vi "TestVision_v2.vi"() -> ()   [LabVIEW 2019]
uses:
  <vilib>/vision/Image Controls.llb/IMAQ Image.ctl
  <vilib>/userDefined/High Color/IMAQdx.ctl
  <vilib>/vision/driver/NI_Vision_Acquisition_Software.lvlib
  <vilib>/vision/NI_Vision_Development_Module.lvlib
panel:
  in  "Image Type":T1 items=["Grayscale (U8)", "Grayscale (I16)", "Grayscale (SGL)", "Complex (CSG)", "RGB (U32)", "HSL (U32)", "RGB (U64)", "Grayscale (U16)"]
  out "Circle Found":bool
  out "Fitted Circle":T2 {"Average SNR (dB)" format="%.2f"; "Average Strength" format="%.2f"; "Roundness (Real-World)" format="%.2f"; "Radius (Real-World)" format="%.2f"; "Center (Real-World)"."Y" format="%.2f"; "Center (Real-World)"."X" format="%.2f"; "Radius (Pixels)" format="%.2f"; "Center (Pixels)"."Y" format="%.2f"; "Center (Pixels)"."X" format="%.2f"}
  out "Image Out":T3
  out "Image 2":T3(plugin-control)
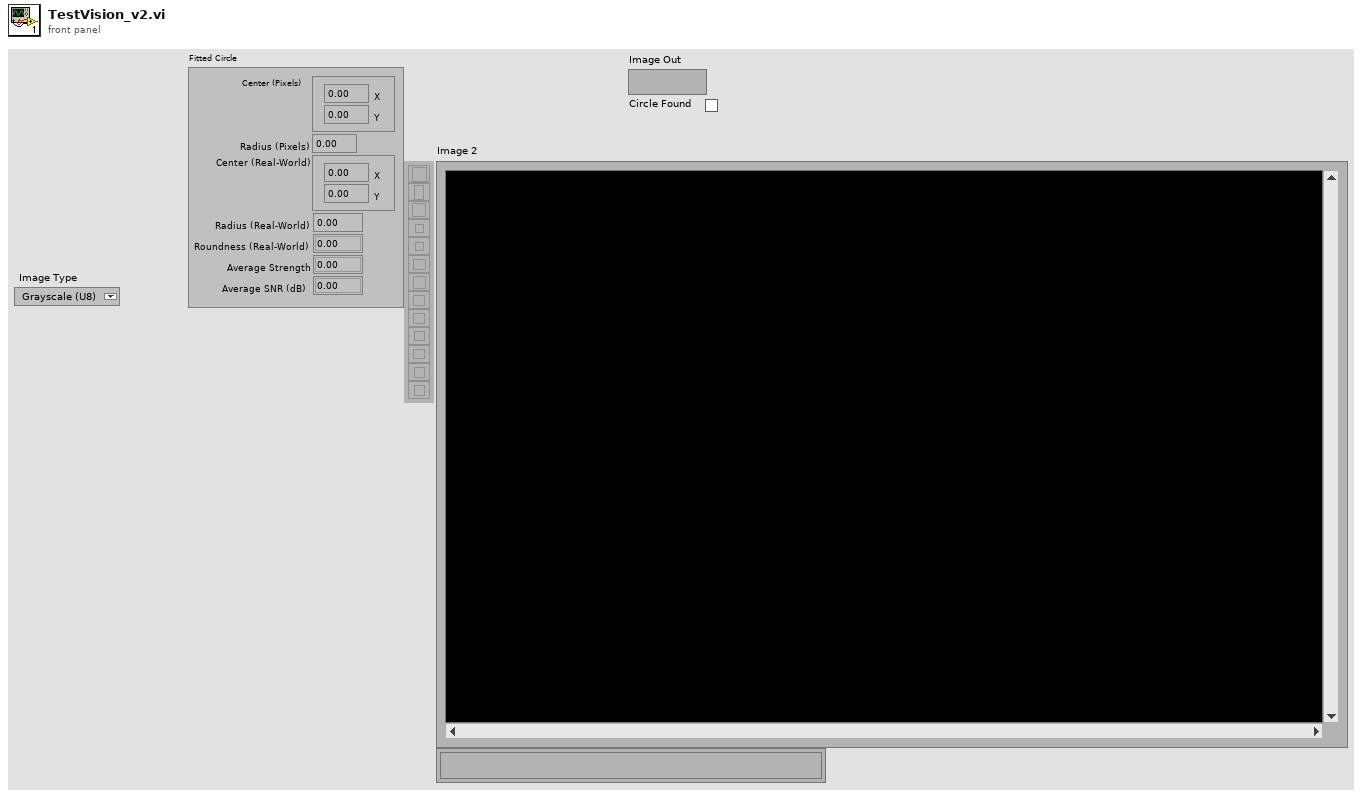
[diagram p1: front panel]
types:
  T1 = typedef "Image Type" = u32
  T2 = cluster{"Center (Pixels)":cluster{"X":sgl, "Y":sgl}, "Radius (Pixels)":dbl, "Center (Real-World)":cluster{"X":sgl, "Y":sgl}, "Radius (Real-World)":dbl, "Roundness (Real-World)":dbl, "Average Strength":dbl, "Average SNR (dB)":dbl}
  T3 = typedef "IMAQ Image.ctl" = refnum<image>
  T4 = typedef "IMAQdx.ctl" = refnum<k21>
  T5 = cluster{"Global Rectangle":i32[], "Contours":cluster{"Contour Type":u32, "ROI Type":u32, "Points":i32[]}[]}
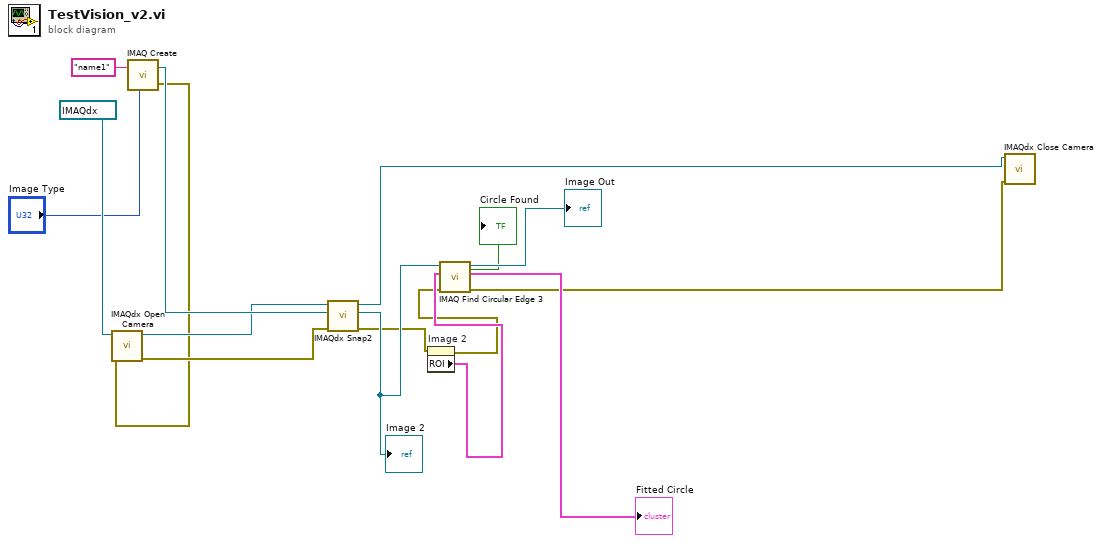
[diagram p0: block diagram]
diagram:
  n1 = call "IMAQ Create"("Image Name"="name1", "Image Type"="Image Type") -> ("New Image"=w13:T3, "error out"=w10:errorcluster)  [unwired: 3 in]
  n2 = call <vilib>:"IMAQdx Open Camera.vi"("error in"=w10, "Session In"=T4 "cam0") -> ("error out"=w14:errorcluster, "Session Out"=w12:T4)  [unwired: 8 in]
  n3 = call <vilib>:"IMAQdx Snap2.vi"("error in"=w14, "Image In"=w13, "Session In"=w12) -> ("error out"=w2:errorcluster, "Image Out"=w9:T3, "Session Out"=w11:T4)  [unwired: 6 in]
  "Image 2" <- w9
  n4 = property on="Image 2" class="ImageControl"(error in=w2) -> (error out=w1:errorcluster, "ROI"=w5:T5)  [unwired: 1 in, 1 out]
  n5 = call "IMAQ Find Circular Edge 3"("error in (no error)"=w1, "ROI Descriptor"=w5, "Image"=w9) -> ("error out"=w4:errorcluster, "Fitted Circle"=→"Fitted Circle":T2, "Image Out"=→"Image Out":T3, "Circle Found"=→"Circle Found":bool)  [unwired: 4 in, 1 out]
  n6 = call <vilib>:"IMAQdx Close Camera.vi"("error in"=w4, "Session In"=w11) -> ()  [unwired: 9 in, 1 out]
